vi "軟體極限.vi"   [LabVIEW 2014]
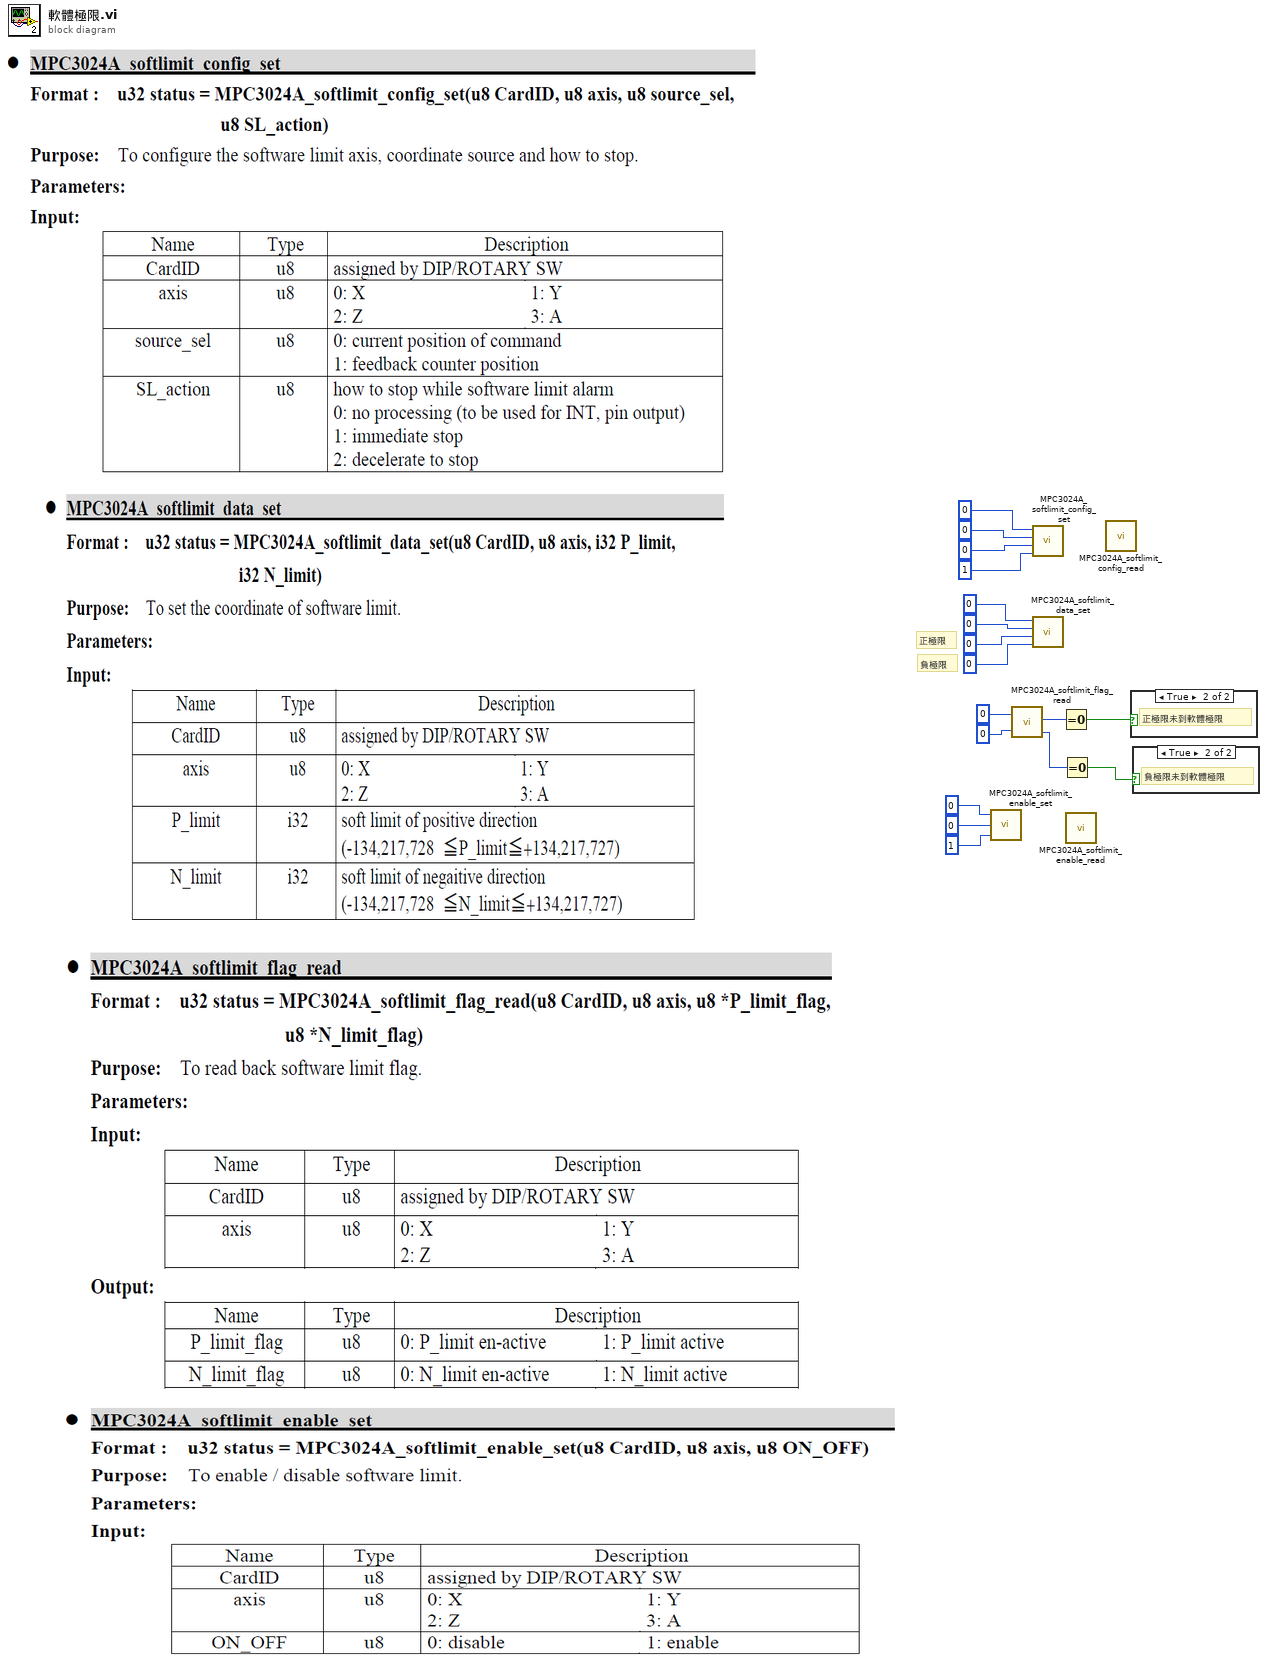
[diagram p0: block diagram]
diagram:
  # "負極限"
  # "正極限"
  n1 = call "MPC3024A_softlimit_enable_set.vi"("ON_OFF"=u8 1, "axis"=u8 0, "CardID"=u8 0) -> ()  [unwired: 1 out]
  n2 = call "MPC3024A_softlimit_flag_read.vi"("CardID"=u8 0, "axis"=u8 0) -> ("P_limit_flag"=w7:u8, "N_limit_flag"=w5:u8)  [unwired: 1 out]
  n3 = call "MPC3024A_softlimit_config_set.vi"("SL_action"=u8 1, "source_sel"=u8 0, "axis"=u8 0, "CardID"=u8 0) -> ()  [unwired: 1 out]
  n4 = call "MPC3024A_softlimit_data_set.vi"("N_limit"=0, "P_limit"=0, "axis"=u8 0, "CardID"=u8 0) -> ()  [unwired: 1 out]
  n5 = Equal To 0?(x=w7) -> (x = 0?=w6:bool)
  n6 = Equal To 0?(x=w5) -> (x = 0?=w4:bool)
  n7 = call "MPC3024A_softlimit_enable_read.vi"() -> ()  [unwired: 2 in, 2 out]
  n8 = call "MPC3024A_softlimit_config_read.vi"() -> ()  [unwired: 2 in, 3 out]
  n9 = case shown="True" w6 {
    frame False {
      # "正極限已到軟體極限"
    }
    frame True {
      # "正極限未到軟體極限"
    }
  }
  n10 = case shown="True" w4 {
    frame False {
      # "負極限已到軟體極限"
    }
    frame True {
      # "負極限未到軟體極限"
    }
  }
